vi "MIMO_RX.vi"() -> ()   [LabVIEW 2012]
uses:
  Synchronizer/Synchronizer.lvclass
  <instrlib>/niUSRP/niUSRP Fetch Rx Data (2D CDB).vi
  Transport Layer/UDP Rx.lvclass
panel:
  in  "ZC-Generation options":T1={"Sequence length"=64, "Sequence Root"=25, "# of subcarriers"=31, "Amplitude"=8.0, "Decimation Factor"=4, "Threshold"=20.0} {"Decimation Factor" min=1 max=8 step=1}
  in  "UDP Config":T2={"Local UDP Port (Tx)"=1002, "Remote IP (Rx)"="localhost", "Remote UDP Port (Rx)"=1234, "Timeout [ms]"=1}
  out "SNR":dbl[][](graph)
  out "Constellation":cluster{dbl[], dbl[]}[](graph)
  out "SNR Pilots (Before Equalizer)":dbl[][](graph)
  out "SNR Pilots (After Equalizer)":dbl[][](graph)
  out "Bit Rate [bps]":dbl=500248.1389578164 format="%#.1p"
  out "Performance [%]":dbl=75.03722084367246 format="%#.1f"
  out "Number of samples\nto receive":i32=16120
  out "Received Packet?":bool
  out "Synch. Detected?":bool
  in  "System options":T3={"Samples per symbol"=6, "Roll-Off"=0.75, "Filter length (symbols)"=3, "Modulation Type"=enum."16-QAM", "Payload Symbols"=1008, "Symbols per Pilot"=6} {"Symbols per Pilot" min=6 max=16 step=2; "Payload Symbols" min=16 max=8192 step=16; "Filter length (symbols)" min=1 max=9 step=2; "Roll-Off" min=0.0 max=1.0 step=0.01; "Samples per symbol" min=2 max=32 step=2}
  out "Peak Position":i32=513
  in  "Rx Parameters":T4={"IQ rate (Hz)"=4000000.0, "Carrier frequency [Hz]"=1187500000.0, "Gain [dB]"=20.0, "Antenna"="TX/RX", "Rx device name"="192.168.10.4; 192.168.10.5;"} {"Gain [dB]" format="%#_6f"; "Carrier frequency [Hz]" format="%#_6p"; "IQ rate (Hz)" format="%#_6p"}
  in  "Stop":bool
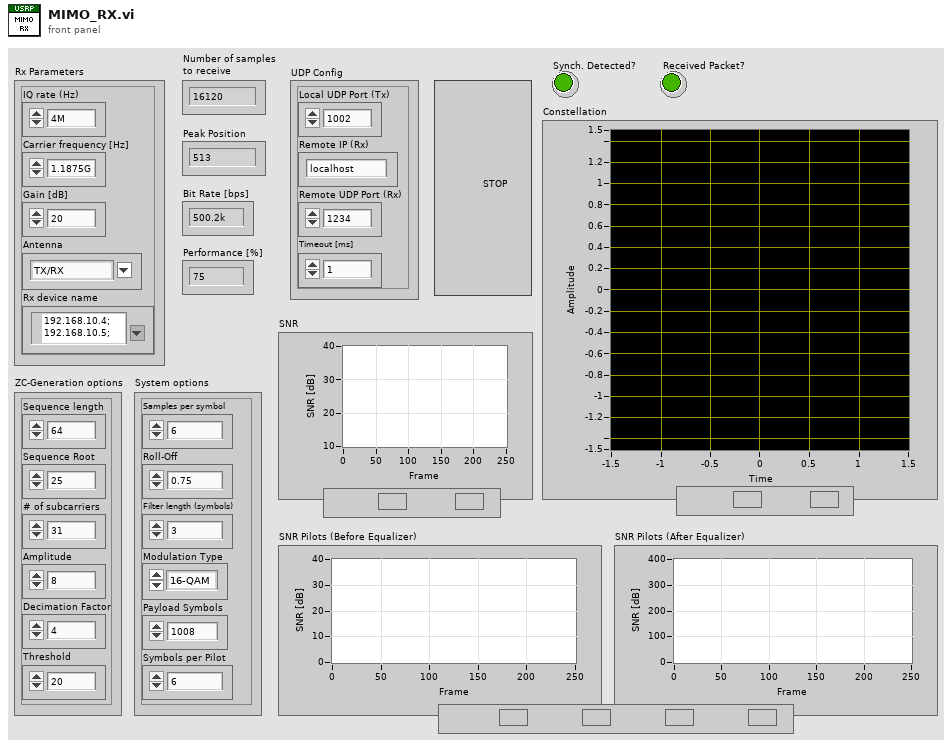
[diagram p1: front panel]
types:
  T1 = cluster{"Sequence length":i32, "Sequence Root":i32, "# of subcarriers":i32, "Amplitude":dbl, "Decimation Factor":u8, "Threshold":dbl}
  T2 = cluster{"Local UDP Port (Tx)":u16, "Remote IP (Rx)":string, "Remote UDP Port (Rx)":u16, "Timeout [ms]":u16}
  T3 = cluster{"Samples per symbol":i32, "Roll-Off":dbl, "Filter length (symbols)":i32, "Modulation Type":enum16{"BPSK", "4-QAM", "16-QAM", "64-QAM"}, "Payload Symbols":i32, "Symbols per Pilot":i32}
  T4 = cluster{"IQ rate (Hz)":dbl, "Carrier frequency [Hz]":dbl, "Gain [dB]":dbl, "Antenna":string, "Rx device name":refnum<k15>}
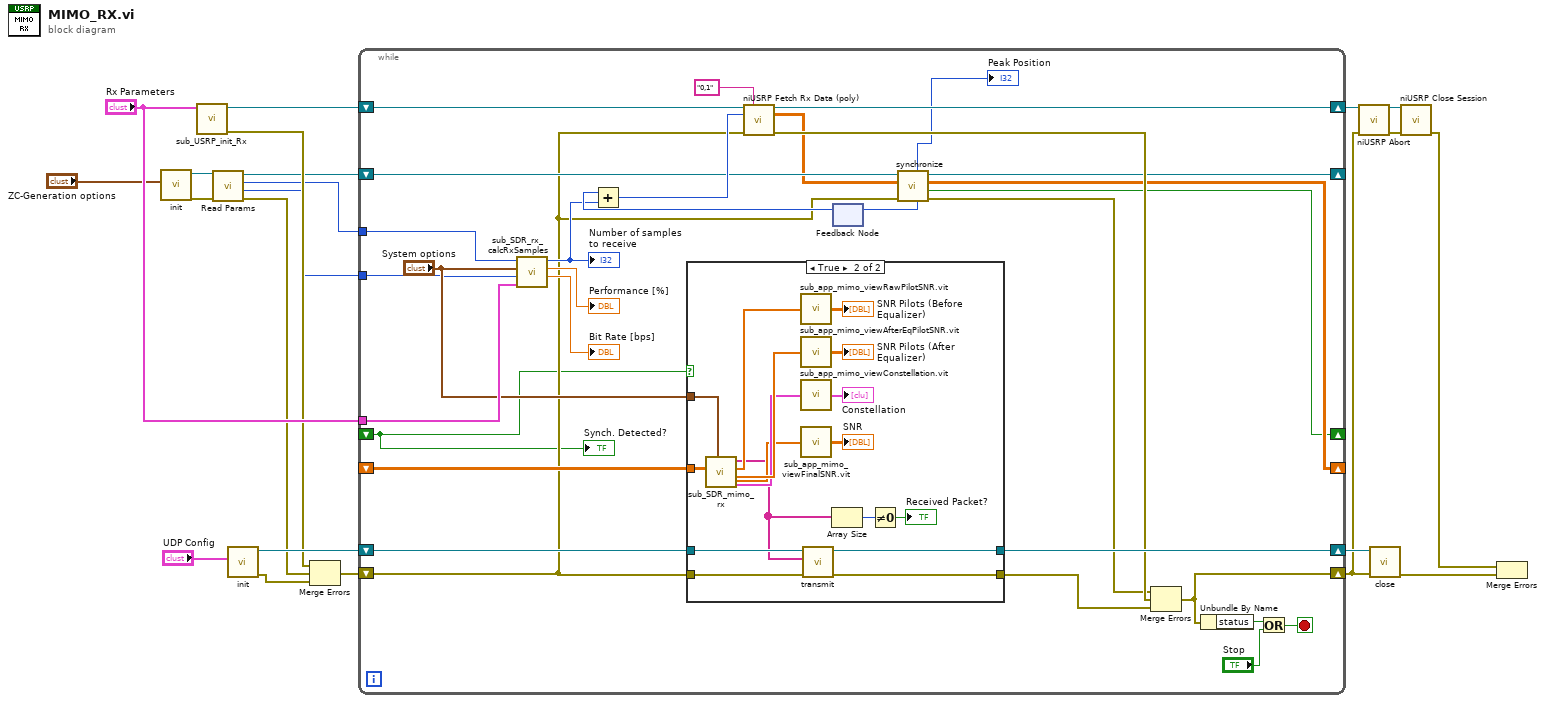
[diagram p0: block diagram]
diagram:
  n1 = call "init.vi"("ZC-Generation options"="ZC-Generation options") -> ("error out"=w1:errorcluster, "Synchronizer out"=w2:refnum<class "Synchronizer.lvclass">)  [unwired: 9 in]
  n2 = call "sub_USRP_init_Rx.vi"("Rx Parameters"="Rx Parameters") -> ("Error out"=w9:errorcluster, "Rx Session handle out"=w21:refnum<k15>)  [unwired: 9 in]
  n3 = call-dynamic "Read Params.vi"("error in (no error)"=w1, "Synchronizer in"=w2) -> ("error out"=w6:errorcluster, "Decimation Factor"=w5:u8, "Sequence length"=w4:i32, "Synchronizer out"=w3:refnum<class "Synchronizer.lvclass">)  [unwired: 6 in]
  n4 = call "init.vi"("UDP Config"="UDP Config") -> ("error out"=w8:errorcluster, "UDP Out"=w15:refnum<class "UDP Rx.lvclass">)  [unwired: 9 in]
  n5 = Merge Errors(w9, w6, w8) -> (w7:errorcluster)
  n6 = while {
    shift-right: [w35] -> w11
    shift-left: w7 -> [w26]
    shift-right: [w47] -> w20
    shift-left: w21 -> [w48]
    tunnel: "Rx Parameters" -> [w40]
    shift-right: [w33] -> _
    shift-left: _ -> [w38]
    shift-right: [w44] -> w14
    shift-left: w15 -> [w37]
    shift-right: [w28] -> _
    shift-left: w3 -> [w31]
    tunnel: w4 -> [w27]
    shift-right: [w24] -> _
    shift-left: _ -> [w23]
    tunnel: w5 -> [w22]
    stop <- w52 stop-if-true
    n7 = call "sub_SDR_rx_calcRxSamples.vi"("Rx Parameters"=w40, "decimating factor"=w22, "System options"="System options", "Synch. Seq. Len"=w27) -> ("Bit Rate [kbps]"=→"Bit Rate [bps]":dbl, "Performance"=→"Performance [%]":dbl, "Numeric"=w43:i32)  [unwired: 5 in]
    "Number of samples\nto receive" <- w43
    n8 = case shown="True" w23 {
      tunnel: w38 -> [_ w71]
      tunnel: "System options" -> [_ w70]
      tunnel: w26 -> [w54 w64]
      tunnel: w37 -> [w53 w63]
      tunnel: [w53 w65] -> w44
      tunnel: [w54 w62] -> w36
      frame False {
      }
      frame True {
        n9 = call "sub_SDR_mimo_rx.vi"("System options"=w70, "Radio Frame"=w71) -> ("Constellation Data"=w67:cluster{dbl[], dbl[]}[], "Pilot SNR After equalization"=w68:dbl[], "SNR Before Equalizer"=w69:dbl[], "Received Packets in current frame"=w55:string[], "Received Data SNR"=w66:dbl[])  [unwired: 5 in]
        n10 = call "sub_app_mimo_viewRawPilotSNR.vit"("SNR Before Equalizer"=w69) -> ("SNR Pilots (Before Equalizer)"=→"SNR Pilots (Before Equalizer)":dbl[][])
        n11 = call "sub_app_mimo_viewAfterEqPilotSNR.vit"("Input values"=w68) -> ("SNR Pilots (After Equalizer)"=→"SNR Pilots (After Equalizer)":dbl[][])
        n12 = call "sub_app_mimo_viewConstellation.vit"("Constellation Data"=w67) -> ("Constellation"=→"Constellation":cluster{dbl[], dbl[]}[])
        n13 = call "sub_app_mimo_viewFinalSNR.vit"("Received Data SNR"=w66) -> ("SNR"=→"SNR":dbl[][])
        n14 = call "transmit.vi"("error in (no error)"=w64, "Packets"=w55, "UDP in"=w63) -> ("error out"=w62:errorcluster, "UDP out"=w65:refnum<class "UDP Rx.lvclass">)  [unwired: 7 in]
        n15 = Array Size(array=w55) -> (size(s)=w57:i32)
        n16 = Not Equal To 0?(x=w57) -> (x != 0?=→"Received Packet?":bool)
      }
    }
    n17 = feedback #1() -> (w45:i32)  [unwired: 1 in]
    n18 = Add(x=w45, y=w43) -> (x+y=w46:i32)
    n19 = call-poly <instrlib>:"niUSRP Fetch Rx Data (poly).vi"("session handle"=w48, "channel list"="0,1", "number of samples"=w46, "error in (no error)"=w26) -> ("session handle out"=w47:refnum<k15>, "data"=w29:cdb[][], "error out"=w34:errorcluster)  [unwired: 8 in, 1 out]
    n20 = call-dynamic "synchronize.vi"("error in (no error)"=w26, "Received frame In"=w29, "Synchronizer in"=w31) -> ("error out"=w30:errorcluster, "Detected?"=w24:bool, "Received frame Out"=w33:cdb[][], "Synchronizer out"=w28:refnum<class "Synchronizer.lvclass">, "NextOffset"=w25:i32, "Peak Position"=→"Peak Position":i32)  [unwired: 3 in]
    n21 = feedback-in #1(w25) -> ()
    n22 = Merge Errors(w30, w34, w36) -> (w35:errorcluster)
    n23 = Unbundle By Name(w35) -> ("status"=w51:bool)
    n24 = Or(x=w51, y="Stop") -> (x .or. y?=w52:bool)
    "Synch. Detected?" <- w23
  }
  n25 = call <instrlib>:"niUSRP Abort.vi"("session handle"=w20, "error in (no error)"=w11) -> ("session handle out"=w19:refnum<k15>, "error out"=w18:errorcluster)  [unwired: 12 in]
  n26 = call "close.vi"("error in (no error)"=w11, "UDP in"=w14) -> ("error out"=w12:errorcluster)  [unwired: 9 in]
  n27 = call <instrlib>:"niUSRP Close Session.vi"("session handle"=w19, "error in (no error)"=w18) -> ("error out"=w13:errorcluster)  [unwired: 13 in]
  n28 = Merge Errors(w13, w12) -> ()  [unwired: 1 out]
